vi "Extract Channel Data.vi"(10 "module configuration in":refnum<class "TBM module configuration.lvclass">, 11 "Engine Configuration":refnum<class "engine configuration.lvclass">) -> (1 "Channel Data":string[][](array[string]))   [LabVIEW 2013, in "fixed channel editor.lvclass"]
uses:
  fixed channel editor.lvclass
  <vilib>/NI/Module Execution Interface/Engine Configuration/engine configuration.lvclass
  <vilib>/NI/Tag Bus Module Framework/module configuration/TBM module configuration.lvclass
  <vilib>/NI/Tag Bus Module Framework/root configuration/TBM configuration.lvclass/TBM configuration.ctl
  <vilib>/NI/Tag Bus/tag/tag descriptor.lvclass/tag descriptor.ctl
  <vilib>/NI/Tag Bus Module Framework/channel/TBM channel.lvclass/TBM channel.ctl
  <vilib>/NI/Tag Bus Module Framework/root configuration/create GUID.vi
  <vilib>/NI/Tag Bus/tag/tag descriptor.lvclass
  <vilib>/NI/Tag Bus Module Framework/root configuration/TBM configuration.lvclass
  <vilib>/NI/Tag Bus Module Framework/channel/TBM channel.lvclass
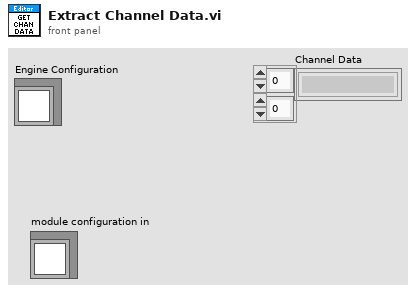
[diagram p1: front panel]
types:
  T1 = typedef "TBM channel.lvclass/channel classification.ctl" = enum16{"input data", "output data", "processing parameter", "processing result"}
  T2 = typedef "tag bus.lvlib/tag descriptor.lvclass/Data Type.ctl" = enum16{"Double", "Single", "I64", "I32", "I16", "I8", "U64", "U32", "U16", "U8", "Boolean", "String", "Array of Double", "Array of Single", "Array of I64", "Array of I32", "Array of I16", "Array of I8", "Array of U64", "Array of U32", "Array of U16", "Array of U8", "Array of Boolean", "Array of String"}
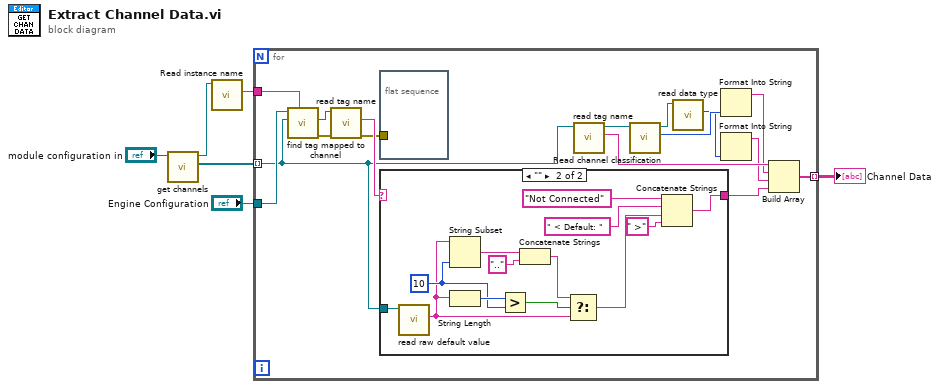
[diagram p0: block diagram]
diagram:
  n1 = call-dynamic "get channels.vi"("module configuration in"="module configuration in") -> ("channels"=w2:refnum<class "TBM channel.lvclass">[], "module configuration out"=w3:refnum<class "TBM module configuration.lvclass">)  [unwired: 9 in]
  n2 = call <vilib>:"Read instance name.vi"("configuration in"=w3) -> ("instance id"=w5:string)  [unwired: 8 in, 2 out]
  n3 = for {
    tunnel: w2 -> [w14] mode=indexing
    tunnel: [w20] -> w6 mode=indexing
    tunnel: w5 -> [w19]
    tunnel: "Engine Configuration" -> [w22]
    n4 = call <vilib>:"find tag mapped to channel.vi"("owner"=w19, "channel"=w14, "engine configuration in"=w22) -> ("error out"=w18:errorcluster, "tag"=w21:refnum<class "tag descriptor.lvclass">)  [unwired: 6 in, 1 out]
    n5 = call <vilib>:"read tag name.vi"("error in"=w18, "system tag in"=w21) -> ("error out"=w15:errorcluster, "name"=w17:string)  [unwired: 7 in, 1 out]
    n6 = flat-sequence {
      tunnel: w15 -> [_]
      frame #0 {
      }
    }
    n7 = case shown="\"\"" w17 {
      selector: w17 -> [w23 _]
      tunnel: [w23 w24] -> w16
      tunnel: w14 -> [_ w26]
      frame Default {
      }
      frame "" {
        w32 = 10 ("y")
        n8 = call <vilib>:"read raw default value.vi"("system tag in"=w26) -> ("raw default"=w28:string)  [unwired: 8 in, 2 out]
        n9 = String Subset(string=w28, length (rest)=w32) -> (substring=w30:string)  [unwired: 1 in]
        n10 = String Length(string=w28) -> (length=w34:i32)
        n11 = Greater?(x=w34, y=w32) -> (0:w33:bool)
        n12 = Concatenate Strings(w30, ".." ("string")) -> (w31:string)
        n13 = Select(t=w31, s=w33, f=w28) -> (s? t:f=w27:string)
        n14 = Concatenate Strings("Not Connected", " < Default: " ("string"), w27, " >" ("string")) -> (w24:string)
      }
    }
    n15 = call <vilib>:"read tag name.vi"("system tag in"=w14) -> ("name"=w13:string, "system tag out"=w7:refnum<class "TBM channel.lvclass">)  [unwired: 8 in, 1 out]
    n16 = call <vilib>:"Read channel classification.vi"("channel in"=w7) -> ("channel classification"=w12:T1, "channel out"=w9:refnum<class "TBM channel.lvclass">)  [unwired: 8 in, 1 out]
    n17 = call <vilib>:"read data type.vi"("system tag in"=w9) -> ("data type"=w8:T2)  [unwired: 8 in, 2 out]
    n18 = Format Into String(w12) -> (resulting string=w11:string)  [unwired: 3 in, 1 out]
    n19 = Format Into String(w8) -> (resulting string=w10:string)  [unwired: 3 in, 1 out]
    n20 = Build Array(w13, w11, w10, w16) -> (w20:string[])
  }
  "Channel Data" <- w6
